vi "Accelerometer Filter for Bumps.vi"(4 "filter factor (0-1)":dbl=0.02, 6 "accelerometer (g)":T2 {"z axis (g)" format="%.3f"; "y axis (g)" format="%.3f"; "x axis (g)" format="%.3f"}) -> (1 "filtered out":T1 {"All Mag" format="%_3f"; "Vert Mag" format="%_3f"; "x axis (g)" format="%_3f"; "y axis (g)" format="%_3f"; "z axis (g)" format="%_3f"; "Horiz Mag" format="%_3f"}, 2 "abs delta":T1 {"All Mag" format="%_3f"; "Vert Mag" format="%_3f"; "x axis (g)" format="%_3f"; "y axis (g)" format="%_3f"; "z axis (g)" format="%_3f"; "Horiz Mag" format="%_3f"})   [LabVIEW 2013]
uses:
  Accelerometer.ctl
  Accel Filtered.ctl
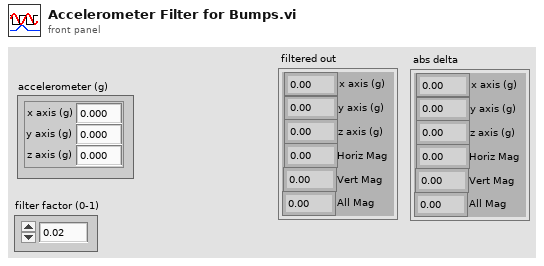
[diagram p1: front panel]
types:
  T1 = typedef "Accel Filtered.ctl" = cluster{"x axis (g)":dbl, "y axis (g)":dbl, "z axis (g)":dbl, "Horiz Mag":dbl, "Vert Mag":dbl, "All Mag":dbl}
  T2 = typedef "Accelerometer.ctl" = cluster{"x axis (g)":dbl, "y axis (g)":dbl, "z axis (g)":dbl}
  T3 = cluster{"[0]":dbl, "[1]":dbl, "[2]":dbl, "[3]":dbl, "[4]":dbl, "[5]":dbl}
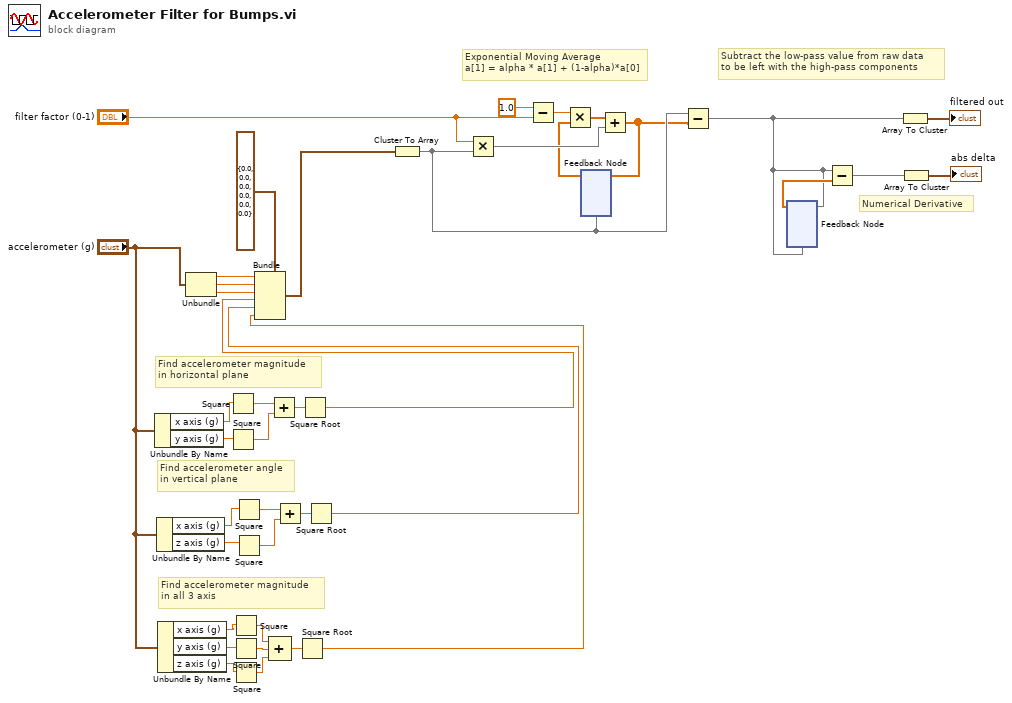
[diagram p0: block diagram]
diagram:
  # "Find accelerometer magnitude\nin all 3 axis"
  # "Find accelerometer angle\nin vertical plane"
  # "Numerical Derivative"
  # "Subtract the low-pass value from raw data\nto be left with the high-pass components"
  # "Find accelerometer magnitude\nin horizontal plane"
  # "Exponential Moving Average\na[1] = alpha * a[1] + (1-alpha)*a[0]"
  n1 = Unbundle By Name("accelerometer (g)") -> ("x axis (g)"=w34:dbl, "y axis (g)"=w33:dbl)
  n2 = Unbundle By Name("accelerometer (g)") -> ("x axis (g)"=w3:dbl, "z axis (g)"=w4:dbl)
  n3 = Unbundle By Name("accelerometer (g)") -> ("x axis (g)"=w19:dbl, "y axis (g)"=w18:dbl, "z axis (g)"=w16:dbl)
  n4 = Unbundle("accelerometer (g)") -> ("x axis (g)"=w24:dbl, "y axis (g)"=w23:dbl, "z axis (g)"=w22:dbl)
  n5 = Square(x=w34) -> (x^2=w31:dbl)
  n6 = Square(x=w33) -> (x^2=w32:dbl)
  n7 = Square(x=w19) -> (x^2=w15:dbl)
  n8 = Square(x=w18) -> (x^2=w14:dbl)
  n9 = Square(x=w16) -> (x^2=w13:dbl)
  n10 = Square(x=w3) -> (x^2=w6:dbl)
  n11 = Square(x=w4) -> (x^2=w5:dbl)
  n12 = Add(x=w31, y=w32) -> (x+y=w30:dbl)
  n13 = Compound Arithmetic op=ADD(w15, w14, w13) -> (w12:dbl)
  n14 = Add(x=w6, y=w5) -> (x+y=w7:dbl)
  n15 = Square Root(x=w12) -> (sqrt(x)=w17:dbl)
  n16 = Square Root(x=w30) -> (sqrt(x)=w8:dbl)
  n17 = Square Root(x=w7) -> (sqrt(x)=w2:dbl)
  n18 = Bundle(cluster=T1 {"x axis (g)"=0.0, "y axis (g)"=0.0, "z axis (g)"=0.0, "Horiz Mag"=0.0, "Vert Mag"=0.0, "All Mag"=0.0}, "x axis (g)"=w24, "y axis (g)"=w23, "z axis (g)"=w22, "Horiz Mag"=w8, "Vert Mag"=w2, "All Mag"=w17) -> (w25:T1)
  n19 = Cluster To Array(cluster=w25) -> (array=w29:dbl[])
  n20 = Multiply(x="filter factor (0-1)", y=w29) -> (x*y=w36:dbl[])
  n21 = Subtract(x=1.0, y="filter factor (0-1)") -> (x-y=w38:dbl)
  n22 = feedback #1(w29) -> (w35:dbl[])
  n23 = Multiply(x=w38, y=w35) -> (x*y=w37:dbl[])
  n24 = Add(x=w37, y=w36) -> (x+y=w28:dbl[])
  n25 = feedback-in #1(w28) -> ()
  n26 = Subtract(x=w29, y=w28) -> (x-y=w21:dbl[])
  n27 = feedback #2(w21) -> (w26:dbl[])
  n28 = feedback-in #2(w21) -> ()
  n29 = Subtract(x=w21, y=w26) -> (x-y=w1:dbl[])
  n30 = Array To Cluster(array=w21) -> (cluster=→"filtered out":T3)
  n31 = Array To Cluster(array=w1) -> (cluster=→"abs delta":T3)
